vi "ELY (SubVI).vi"(8 "error in (no error)":errorcluster, 10 "Electrolizador":string, 11 "Refnum in":T1) -> (0 "error out":errorcluster, 1 "Warning":u16, 2 "Error":u16, 3 "Refnum out":T1, 4 "StartStop":u16, 5 "Produccion":map{string, dbl}(c390), 6 "Medidas":map{string, dbl}(c390), 7 "Estado":u16)   [LabVIEW 2024]
uses:
  <vilib>/OPCUA/controls/OPC UA Client Refnum.ctl
  <vilib>/OPCUA/controls/NodeIds.ctl
  <vilib>/OPCUA/controls/NodeId.ctl
  <vilib>/OPCUA/client/Multiple Read UInt16.vi
  <vilib>/OPCUA/client/Multiple Read Float.vi
  <vilib>/OPCUA/NI OPC UA Client.lvlib
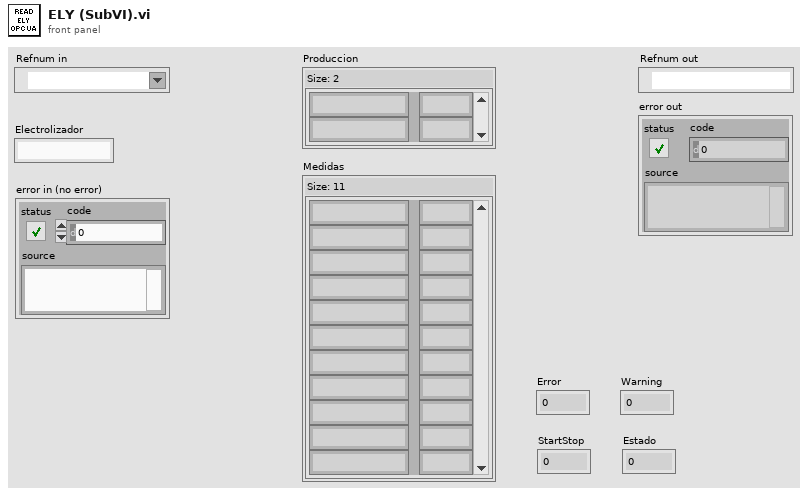
[diagram p1: front panel]
types:
  T1 = typedef "OPC UA Client Refnum.ctl" = refnum<k21>
  T2 = typedef "NodeIds.ctl" = T3[]
  T3 = typedef "NodeId.ctl" = string
  T4 = typedef "OPC UA StatusCode.ctl" = u32
  T5 = cluster{"node ID":T3, "value ":u16, "timestamp":timestamp, "status":T4}[]
  T6 = cluster{"node ID":T3, "value ":sgl, "timestamp":timestamp, "status":T4}[]
  T7 = cluster{"node ID":T3, "value ":u16, "timestamp":timestamp, "status":T4}
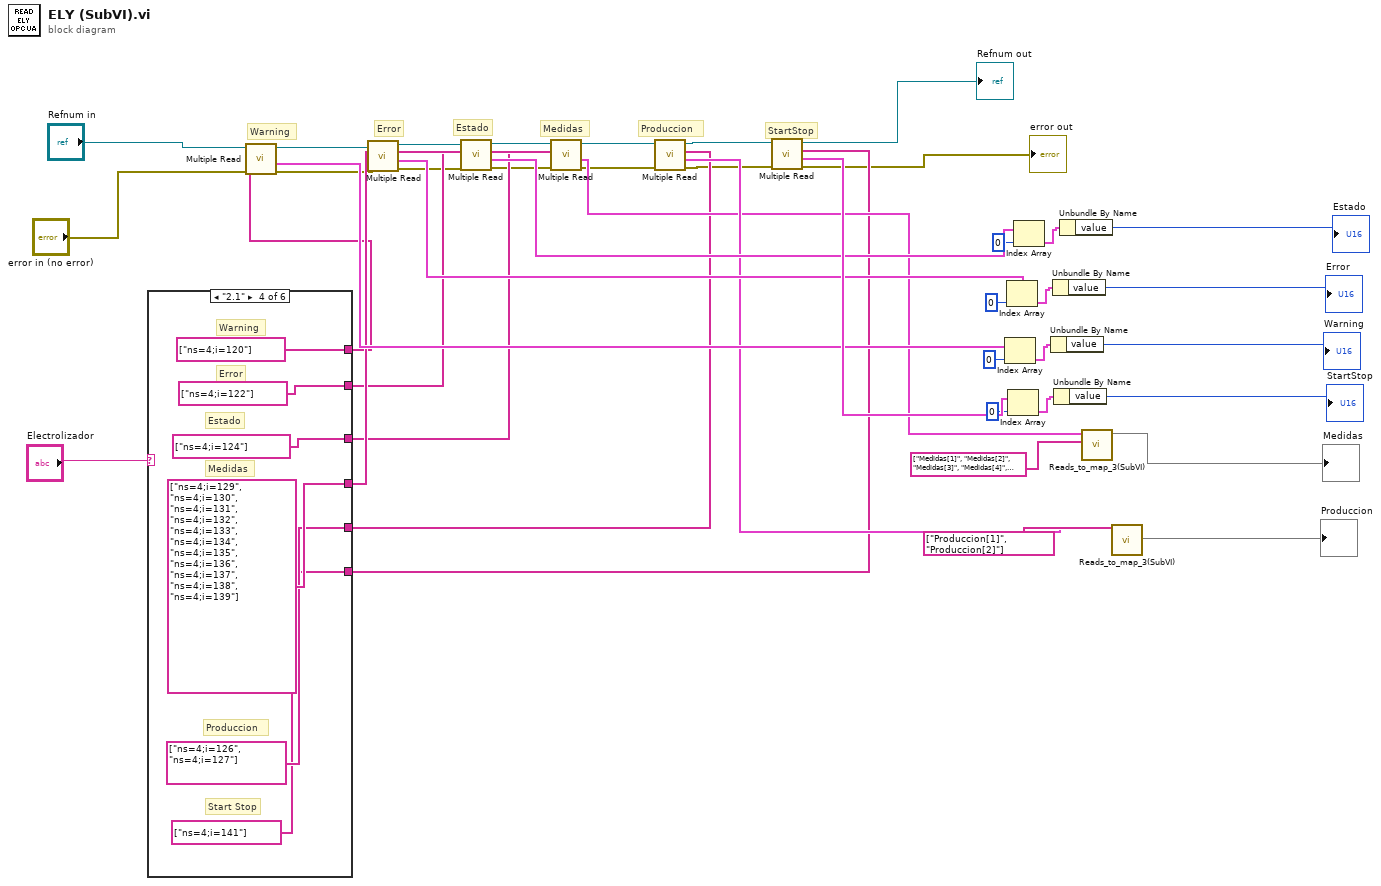
[diagram p0: block diagram]
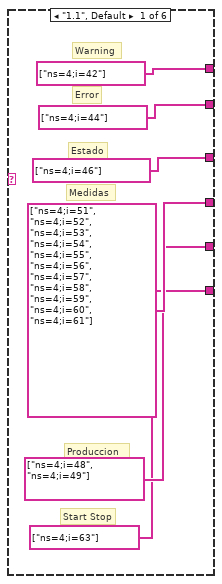
[diagram p2: hidden frame]
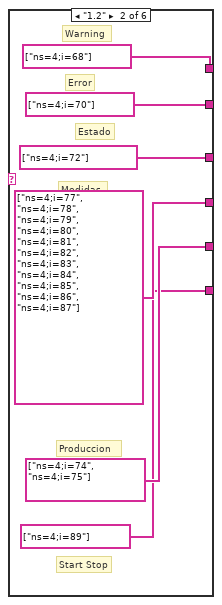
[diagram p3: hidden frame]
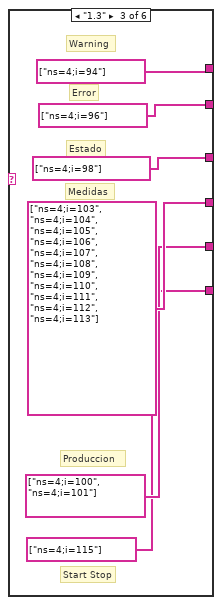
[diagram p4: hidden frame]
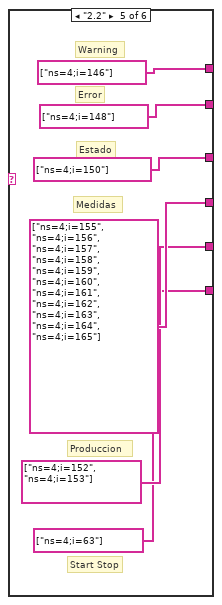
[diagram p5: hidden frame]
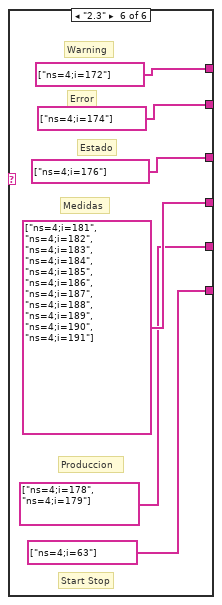
[diagram p6: hidden frame]
diagram:
  # "StartStop"
  # "Produccion"
  # "Medidas"
  # "Estado"
  # "Error"
  # "Warning"
  n1 = case shown="\"2.1\"" "Electrolizador" {
    tunnel: [T2 ["ns=4;i=42"] ("node IDs") T2 ["ns=4;i=68"] ("node IDs") T2 ["ns=4;i=94"] ("node IDs") T2 ["ns=4;i=120"] ("node IDs") T2 ["ns=4;i=146"] ("node IDs") T2 ["ns=4;i=172"] ("node IDs")] -> w15
    tunnel: [T2 ["ns=4;i=44"] ("node IDs") T2 ["ns=4;i=70"] ("node IDs") T2 ["ns=4;i=96"] ("node IDs") T2 ["ns=4;i=122"] ("node IDs") T2 ["ns=4;i=148"] ("node IDs") T2 ["ns=4;i=174"] ("node IDs")] -> w16
    tunnel: [T2 ["ns=4;i=46"] ("node IDs") T2 ["ns=4;i=72"] ("node IDs") T2 ["ns=4;i=98"] ("node IDs") T2 ["ns=4;i=124"] ("node IDs") T2 ["ns=4;i=150"] ("node IDs") T2 ["ns=4;i=176"] ("node IDs")] -> w17
    tunnel: [T2 ["ns=4;i=51", "ns=4;i=52", "ns=4;i=53", "ns=4;i=54", "ns=4;i=55", "ns=4;i=56", "ns=4;i=57", "ns=4;i=58", "ns=4;i=59", "ns=4;i=60", "ns=4;i=61"] ("node IDs") T2 ["ns=4;i=77", "ns=4;i=78", "ns=4;i=79", "ns=4;i=80", "ns=4;i=81", "ns=4;i=82", "ns=4;i=83", "ns=4;i=84", "ns=4;i=85", "ns=4;i=86", "ns=4;i=87"] ("node IDs") T2 ["ns=4;i=103", "ns=4;i=104", "ns=4;i=105", "ns=4;i=106", "ns=4;i=107", "ns=4;i=108", "ns=4;i=109", "ns=4;i=110", "ns=4;i=111", "ns=4;i=112", "ns=4;i=113"] ("node IDs") T2 ["ns=4;i=129", "ns=4;i=130", "ns=4;i=131", "ns=4;i=132", "ns=4;i=133", "ns=4;i=134", "ns=4;i=135", "ns=4;i=136", "ns=4;i=137", "ns=4;i=138", "ns=4;i=139"] ("node IDs") T2 ["ns=4;i=155", "ns=4;i=156", "ns=4;i=157", "ns=4;i=158", "ns=4;i=159", "ns=4;i=160", "ns=4;i=161", "ns=4;i=162", "ns=4;i=163", "ns=4;i=164", "ns=4;i=165"] ("node IDs") T2 ["ns=4;i=181", "ns=4;i=182", "ns=4;i=183", "ns=4;i=184", "ns=4;i=185", "ns=4;i=186", "ns=4;i=187", "ns=4;i=188", "ns=4;i=189", "ns=4;i=190", "ns=4;i=191"] ("node IDs")] -> w18
    tunnel: [T2 ["ns=4;i=48", "ns=4;i=49"] ("node IDs") T2 ["ns=4;i=74", "ns=4;i=75"] ("node IDs") T2 ["ns=4;i=100", "ns=4;i=101"] ("node IDs") T2 ["ns=4;i=126", "ns=4;i=127"] ("node IDs") T2 ["ns=4;i=152", "ns=4;i=153"] ("node IDs") T2 ["ns=4;i=178", "ns=4;i=179"] ("node IDs")] -> w19
    tunnel: [T2 ["ns=4;i=63"] ("node IDs") T2 ["ns=4;i=89"] ("node IDs") T2 ["ns=4;i=115"] ("node IDs") T2 ["ns=4;i=141"] ("node IDs") T2 ["ns=4;i=63"] ("node IDs") T2 ["ns=4;i=63"] ("node IDs")] -> w20
    frame "1.1", Default {
      # "Medidas"
      # "Start Stop"
      # "Produccion"
      # "Estado"
      # "Error"
      # "Warning"
    }
    frame "1.2" {
      # "Medidas"
      # "Start Stop"
      # "Produccion"
      # "Estado"
      # "Error"
      # "Warning"
    }
    frame "1.3" {
      # "Medidas"
      # "Start Stop"
      # "Produccion"
      # "Estado"
      # "Error"
      # "Warning"
    }
    frame "2.1" {
      # "Medidas"
      # "Start Stop"
      # "Produccion"
      # "Estado"
      # "Error"
      # "Warning"
    }
    frame "2.2" {
      # "Medidas"
      # "Start Stop"
      # "Produccion"
      # "Estado"
      # "Error"
      # "Warning"
    }
    frame "2.3" {
      # "Medidas"
      # "Start Stop"
      # "Produccion"
      # "Estado"
      # "Error"
      # "Warning"
    }
  }
  n2 = call-poly <vilib>:"Multiple Read.vi"("error in (no error)"="error in (no error)", "node IDs"=w15, "OPC UA client refnum in"="Refnum in") -> ("error out"=w4:errorcluster, "results"=w27:T5, "OPC UA client refnum out"=w3:T1)  [unwired: 5 in, 1 out]
  n3 = call-poly <vilib>:"Multiple Read.vi"("error in (no error)"=w4, "node IDs"=w16, "OPC UA client refnum in"=w3) -> ("error out"=w6:errorcluster, "results"=w38:T5, "OPC UA client refnum out"=w5:T1)  [unwired: 5 in, 1 out]
  n4 = call-poly <vilib>:"Multiple Read.vi"("error in (no error)"=w6, "node IDs"=w17, "OPC UA client refnum in"=w5) -> ("error out"=w8:errorcluster, "results"=w37:T5, "OPC UA client refnum out"=w7:T1)  [unwired: 5 in, 1 out]
  n5 = call-poly <vilib>:"Multiple Read.vi"("error in (no error)"=w8, "node IDs"=w18, "OPC UA client refnum in"=w7) -> ("error out"=w10:errorcluster, "results"=w22:T6, "OPC UA client refnum out"=w9:T1)  [unwired: 5 in, 1 out]
  n6 = call-poly <vilib>:"Multiple Read.vi"("error in (no error)"=w10, "node IDs"=w19, "OPC UA client refnum in"=w9) -> ("error out"=w12:errorcluster, "results"=w24:T6, "OPC UA client refnum out"=w11:T1)  [unwired: 5 in, 1 out]
  n7 = call-poly <vilib>:"Multiple Read.vi"("error in (no error)"=w12, "node IDs"=w20, "OPC UA client refnum in"=w11) -> ("error out"=→"error out":errorcluster, "results"=w42:T5, "OPC UA client refnum out"=→"Refnum out":T1)  [unwired: 5 in, 1 out]
  n8 = Index Array(array=w27, index=0) -> (element=w29:T7)
  n9 = Index Array(array=w38, index=0) -> (element=w32:T7)
  n10 = Index Array(array=w42, index=0) -> (element=w40:T7)
  n11 = Index Array(array=w37, index=0) -> (element=w35:T7)
  n12 = Unbundle By Name(w29) -> ("value"=→"Warning":u16)
  n13 = Unbundle By Name(w32) -> ("value"=→"Error":u16)
  n14 = Unbundle By Name(w40) -> ("value"=→"StartStop":u16)
  n15 = Unbundle By Name(w35) -> ("value"=→"Estado":u16)
  n16 = call "Reads_to_map_3(SubVI).vi"("Array"=string[] ["Medidas[1]", "Medidas[2]", "Medidas[3]", "Medidas[4]", "Medidas[5]", "Medidas[6]", "Medidas[7]", "Medidas[8]", "Medidas[9]", "Medidas[10]", "Medidas[11]"], "results"=w22) -> ("Map"=→"Medidas":map{string, dbl})  [unwired: 9 in]
  n17 = call "Reads_to_map_3(SubVI).vi"("Array"=string[] ["Produccion[1]", "Produccion[2]"], "results"=w24) -> ("Map"=→"Produccion":map{string, dbl})  [unwired: 9 in]
